vi "Actor Core.vi"(8 "error in":errorcluster, 11 "Pulse Recorder in":refnum<class "NI-Scope Lock-in.lvclass">) -> (0 "error out":errorcluster, 3 "Actor out":refnum<class "Actor.lvclass">)   [LabVIEW 2016, in "NI-Scope Lock-in.lvclass"]
doc: "(<B>Filename</B>: Actor Framework.lvlib:Actor.lvclass:Actor Core.vi)\n\nReceives messages to the actor, reacts to them, and initiates any error handling that may shut the actor down.\n\nDescendant classes may override this VI to append parallel tasks for the actor to complete while it handles messages. Overrides use the Call Parent Method node."
uses:
  NI-Scope Lock-in.lvclass
  <vilib>/ActorFramework/Actor/Actor.lvclass
  NHMFL_Core/Libraries/NI-DAQ/NI-Scope Lock-in Driver/NI-Scope Lock-in Configuration.ctl
  NHMFL_Core/Libraries/Instruments/Pulse Driver/Pusle Driver Configuration.ctl
  Pulse Recorders/Pulse Recorder/Pulse Recorder.lvclass
panel:
  out "Armed":bool
  out "Name":string
  in  "Configuration":T1={"Pulse Configuration"={"Pre-trigger duration"=0.01, "Post-trigger duration"=0.1, "Rate"=1000000.0, "Ranges"=[10.0], "Re-name channels"=[], "Active channels"="0:1", "External clock"=FALSE}, "Points per sine wave"=0} {"Pulse Configuration"."Rate" format="%#_8pHz"; "Pulse Configuration"."Post-trigger duration" format="%#_6ps"; "Pulse Configuration"."Pre-trigger duration" format="%#_6ps"; "Pulse Configuration"."Ranges" format="%#_6pV"}
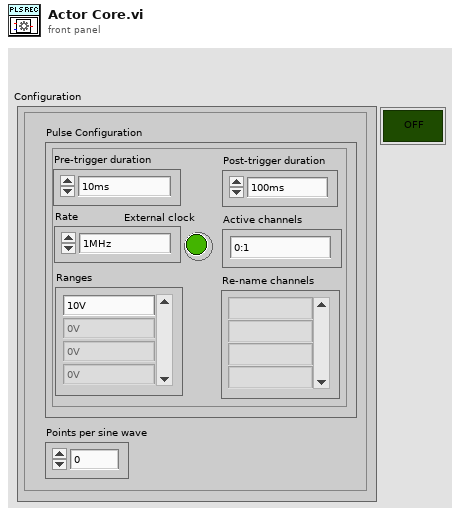
[diagram p1: front panel]
types:
  T1 = typedef "NI-Scope Lock-in Configuration.ctl" = cluster{"Pulse Configuration":T2, "Points per sine wave":i32}
  T2 = typedef "Pusle Driver Configuration.ctl" = cluster{"Pre-trigger duration":dbl, "Post-trigger duration":dbl, "Rate":dbl, "Ranges":dbl[], "Re-name channels":string[], "Active channels":string, "External clock":bool}
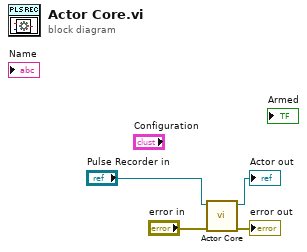
[diagram p0: block diagram]
diagram:
  n1 = call-parent "Actor Core.vi"("error in"="error in", "Pulse Recorder in"="Pulse Recorder in") -> ("error out"=→"error out":errorcluster, "Actor out"=→"Actor out":refnum<class "Actor.lvclass">)  [unwired: 8 in]
